vi "Error Query.vi"(0 "VISA resource name":refnum<visa-resource-name>, 11 "error in (no error)":errorcluster) -> (4 "VISA resource name out":refnum<visa-resource-name>, 6 "Error Code":i32, 8 "Error Message":string, 15 "error out":errorcluster)   [LabVIEW 2016, in "eec EST 300.lvlib"]
doc: "Queries the instrument for any errors in the instrument's error queue. It will continue to read errors until all errors have been read from the instrument. Any errors will be returned in the <B>error out</B> control.\n\n<B>Note:</B>\nThis VI is called automatically by most driver VIs so it is not usually necessary to call this in an application."
uses:
  <instrlib>/eec EST 300/eec EST 300.lvlib
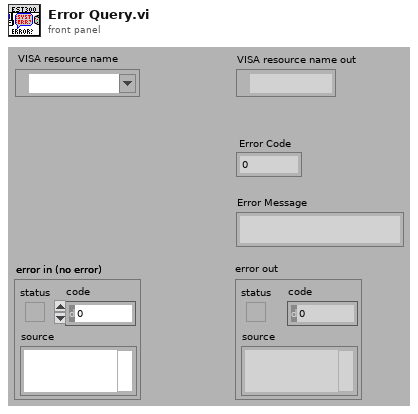
[diagram p1: front panel]
types:
  T1 = cluster{"Operation Complete":bool, "Not Used":bool, "Query Error":bool, "Device Error":bool, "Execution Error":bool, "Command Error":bool, "Not Used":bool, "Power On":bool}
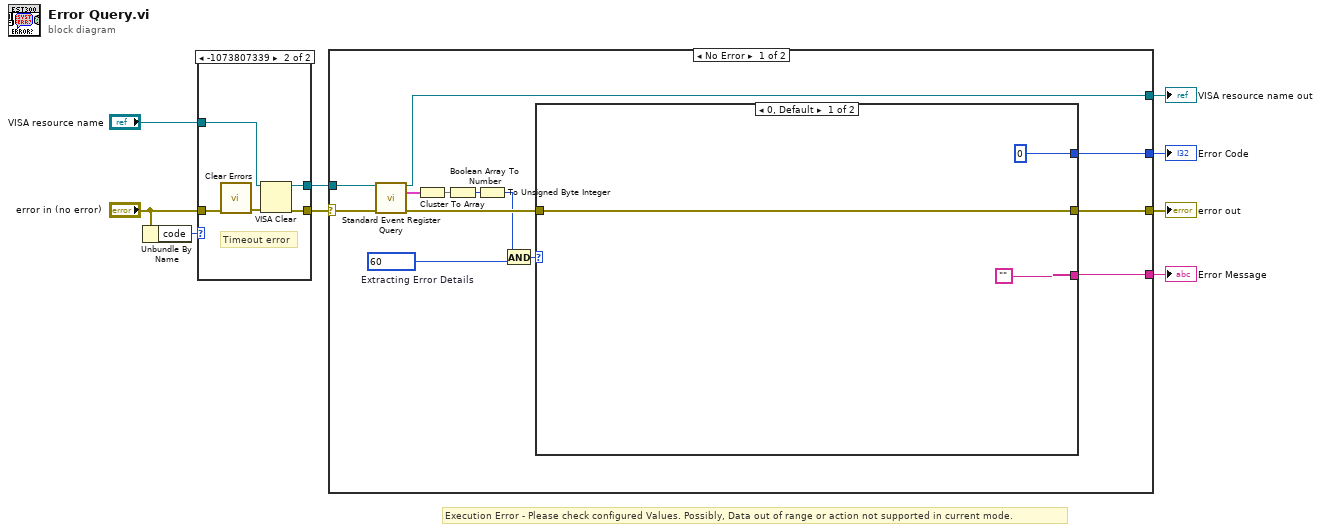
[diagram p0: block diagram]
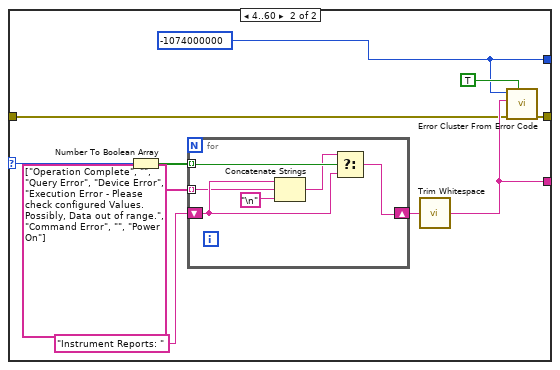
[diagram p2: hidden frame]
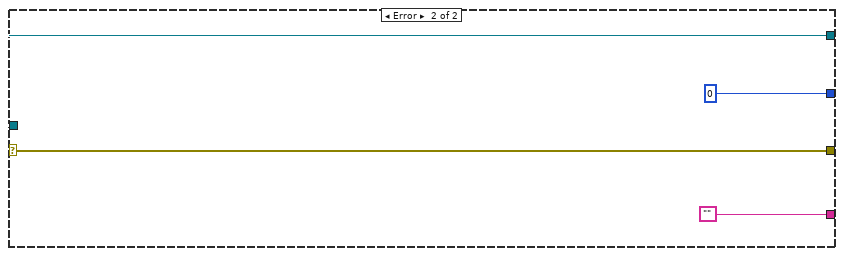
[diagram p3: hidden frame]
diagram:
  # "Execution Error - Please check configured Values. Possibly, Data out of range or action not supported in current mode."
  n1 = Unbundle By Name("error in (no error)") -> ("code"=w3:i32)
  n2 = case shown="-1073807339" w3 {
    tunnel: "error in (no error)" -> [w11 w16]
    tunnel: "VISA resource name" -> [w10 w14]
    tunnel: [w11 w12] -> w4
    tunnel: [w10 w15] -> w5
    frame Default {
    }
    frame -1073807339 {
      # "Timeout error"
      n3 = call <vilib>:"Clear Errors.vi"("error in (no error)"=w16) -> ("error out"=w13:errorcluster)  [unwired: 5 in, 1 out]
      n4 = VISA Clear(VISA resource name=w14, error in (no error)=w13) -> (VISA resource name out=w15:refnum<visa-resource-name>, error out=w12:errorcluster)
    }
  }
  n5 = case shown="No Error" w4 {
    selector: w4 -> [w26 w52]
    tunnel: [w29 w51] -> w9
    tunnel: [w28 w52] -> w8
    tunnel: w5 -> [w27 w51]
    tunnel: [w25 "" ("Empty String Constant")] -> w2
    tunnel: [w24 0 ("Code")] -> w1
    frame No Error {
      w22 = u8 60  # Extracting Error Details
      n6 = call <instrlib>:"Standard Event Register Query.vi"("VISA resource name"=w27, "error in (no error)"=w26) -> ("VISA resource name out"=w29:refnum<visa-resource-name>, "Standard Event Register"=w19:T1, "error out"=w23:errorcluster)  [unwired: 11 in]
      n7 = Cluster To Array(cluster=w19) -> (array=w17:bool[])
      n8 = Boolean Array To Number(Boolean array=w17) -> (number=w18:u32)
      n9 = To Unsigned Byte Integer(number=w18) -> (unsigned 8bit integer=w21:u8)
      n10 = And(x=w21, y=w22) -> (x .and. y?=w20:u8)
      n11 = case shown="0, Default" w20 {
        selector: w20 -> [_ w37]
        tunnel: [w32 w36] -> w28
        tunnel: w23 -> [w32 w34]
        tunnel: ["" ("Empty String Constant") w35] -> w25
        tunnel: [0 ("Code") w33] -> w24
        frame 0, Default {
        }
        frame 4..60 {
          w33 = -1074000000 ("Code")
          n12 = Number To Boolean Array(number=w37) -> (Boolean array=w41:bool[])
          n13 = for {
            tunnel: w41 -> [w48] mode=indexing
            tunnel: string[] ["Operation Complete", "", "Query Error", "Device Error", "Execution Error - Please check configured Values. Possibly, Data out of range.", "Command Error", "", "Power On"] -> [w45] mode=indexing
            shift-right: [w47] -> w39
            shift-left: "Instrument Reports: " -> [w46]
            n14 = Concatenate Strings(w46, w45, "\n" ("Line Feed Constant")) -> (w44:string)
            n15 = Select(t=w44, s=w48, f=w46) -> (s? t:f=w47:string)
          }
          n16 = call <vilib>:"Trim Whitespace.vi"("string"=w39) -> ("trimmed string"=w35:string)  [unwired: 1 in]
          n17 = call <vilib>:"Error Cluster From Error Code.vi"("show call chain? (False)"=TRUE, "error in (no error)"=w34, "error message (\"\")"=w35, "error code (0)"=w33) -> ("error out"=w36:errorcluster)  [unwired: 5 in]
        }
      }
    }
    frame Error {
    }
  }
  "VISA resource name out" <- w9
  "error out" <- w8
  "Error Message" <- w2
  "Error Code" <- w1
